vi "DisplayConsole_Main.vi"(8 "error in (no error)":errorcluster) -> (0 "error out":errorcluster)   [LabVIEW 2017]
doc: "This is Top Level VI for Display Console Module. You can communicate with this module using its API. Communication is made based on queue. This module has not User Interface so I chase State Machine architecture."
uses:
  General/Controls/#TD_General_CommunicationQueueStates_Enum.ctl
  Private controls/#TD_DisplayConsole_InnerData_Cluster.ctl
  Private controls/#TD_DisplayConsole_ModuleStates_Enum.ctl
  Private controls/#TD_DisplayConsole_ModuleData_Cluster.ctl
  General/Controls/#TD_General_FromWho_Enum.ctl
panel:
  out "CardRead":bool caption="Card Read"
  out "MessageScreen":string caption="Message Screen"
  out "CurrentTransaction":string caption="Current Transaction"
  # "[Covers: UI3]"
  # "[Covers: UI3A] \n[Covers: UI3B] \n[Covers: UI3C]"
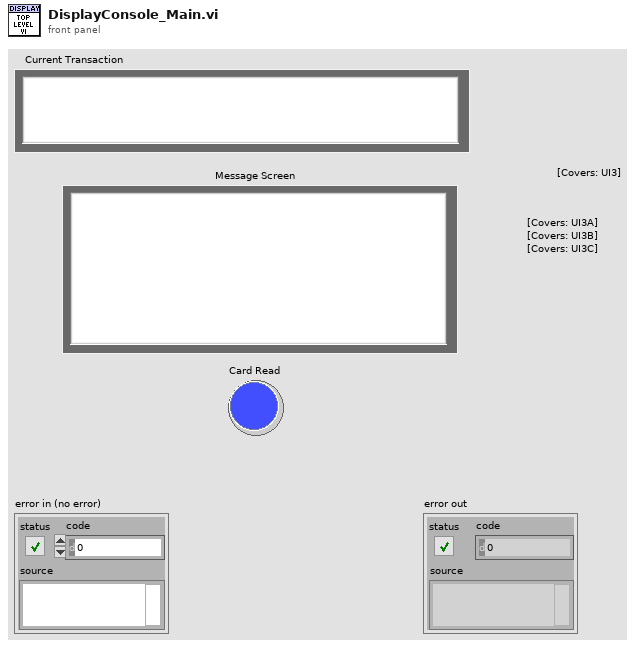
[diagram p1: front panel]
types:
  T1 = typedef "#TD_General_CommunicationQueueStates_Enum.ctl" = enum16{"ERROR_Default", "Obtain", "GetRef", "Enqueue", "EnqueueAtOpp", "GetStatus", "Release"}
  T2 = typedef "#TD_General_FromWho_Enum.ctl" = enum16{"ERROR_Default", "UserConsole", "DisplayConsole", "SensorInterface", "Controller", "Database", "Timing", "AdditionalModule", "ErrorHandling"}
  T3 = typedef "#TD_DisplayConsole_ModuleStates_Enum.ctl" = enum16{"ERROR_Default", "Init", "Close", "ErrorHandling", "UpdateCurrTrans", "UpdateMessage", "NewState", "UpdateCardRead"}
  T4 = typedef "#TD_DisplayConsole_ModuleData_Cluster.ctl" = cluster{"Action":T3, "Data":variant}
  T5 = typedef "#TD_General_IntermoduleData_Cluster.ctl" = cluster{"Sender":T2, "ModuleData":variant}
  T6 = typedef "#TD_DisplayConsole_InnerData_Cluster.ctl" = cluster{"Sth":bool, "CurrentTrans":string, "CardRead":bool, "Messages":string[], "NumericTestAK":dbl}
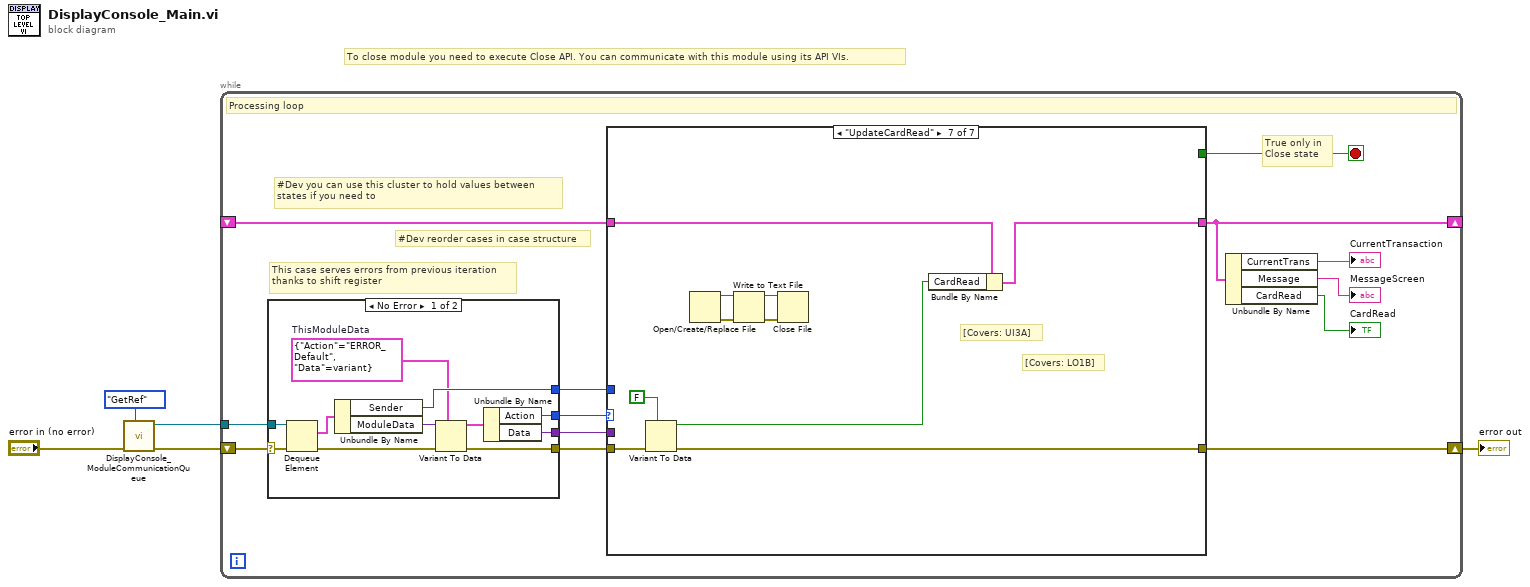
[diagram p0: block diagram]
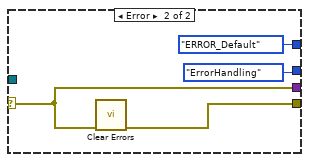
[diagram p2: hidden frame]
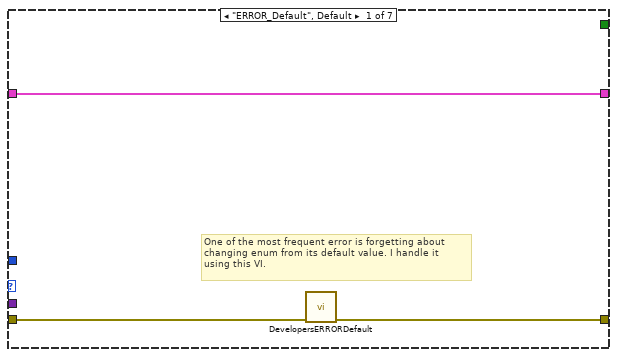
[diagram p3: hidden frame]
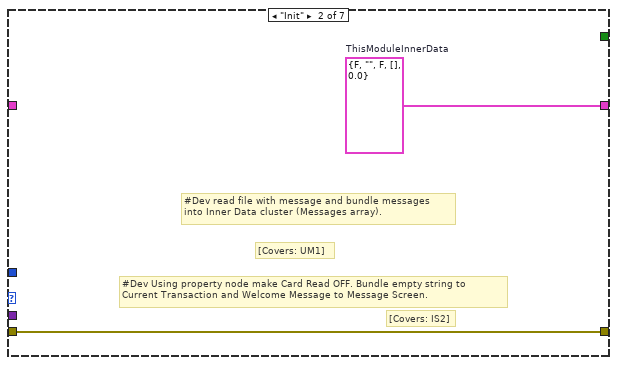
[diagram p4: hidden frame]
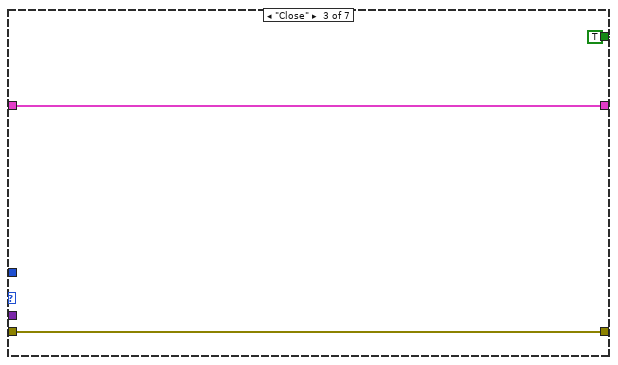
[diagram p5: hidden frame]
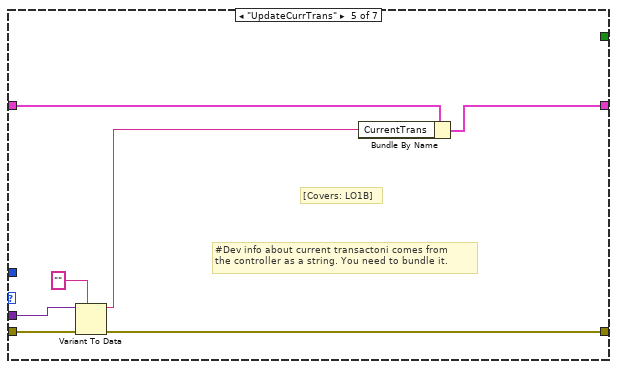
[diagram p7: hidden frame]
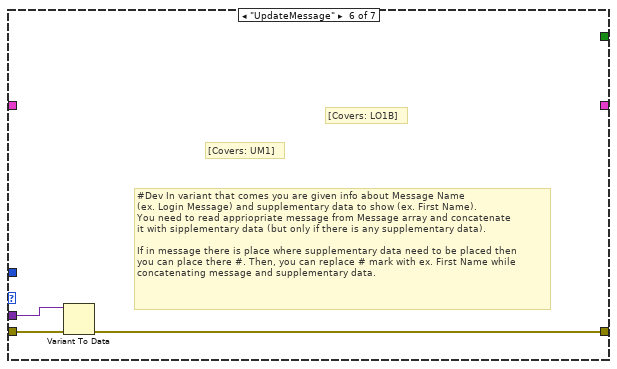
[diagram p8: hidden frame]
diagram:
  # "To close module you need to execute Close API. You can communicate with this module using its API VIs."
  n1 = call "DisplayConsole_ModuleCommunicationQueue.vi"("Action"=#TD_General_CommunicationQueueStates_Enum."GetRef", "error in (no error)"="error in (no error)") -> ("error out"=w2:errorcluster, "Ref out"=w3:refnum<queue>)  [unwired: 7 in, 1 out]
  n2 = while {
    tunnel: w3 -> [w17]
    shift-right: [w11] -> w1
    shift-left: w2 -> [w18]
    shift-right: [w9] -> _
    shift-left: _ -> [w16]
    stop <- w10 stop-if-true
    # "#Dev reorder cases in case structure"
    # "True only in \nClose state"
    # "#Dev you can use this cluster to hold values between \nstates if you need to"
    # "This case serves errors from previous iteration \nthanks to shift register"
    # "Processing loop"
    n3 = case shown="No Error" w18 {
      selector: w18 -> [w29 w33]
      tunnel: w17 -> [w28 _]
      tunnel: [w24 #TD_General_FromWho_Enum."ERROR_Default" ("Sender")] -> w15
      tunnel: [w21 #TD_DisplayConsole_ModuleStates_Enum."ErrorHandling" ("Action")] -> w14
      tunnel: [w20 w33] -> w13
      tunnel: [w19 w32] -> w12
      frame No Error {
        w23 = T4 {"Action"=enum."ERROR_Default", "Data"=variant}  # ThisModuleData
        n4 = Dequeue Element(queue=w28, error in (no error)=w29) -> (element=w27:T5, error out=w25:errorcluster)  [unwired: 1 in, 2 out]
        n5 = Unbundle By Name(w27) -> ("Sender"=w24:T2, "ModuleData"=w26:variant)
        n6 = Variant To Data(error in=w25, type=w23, Variant=w26) -> (data=w22:T4, error out=w19:errorcluster)
        n7 = Unbundle By Name(w22) -> ("Action"=w21:T3, "Data"=w20:variant)
      }
      frame Error {
        n8 = call <vilib>:"Clear Errors.vi"("error in (no error)"=w33) -> ("error out"=w32:errorcluster)  [unwired: 5 in, 1 out]
      }
    }
    n9 = case shown="\"UpdateCardRead\"" w14 {
      tunnel: [w36 w38 w40 w43 w47 _ w60] -> w9
      tunnel: w16 -> [w36 _ w40 w43 w48 _ w61]
      tunnel: w15 -> [_ _ _ _ _ _ _]
      tunnel: w13 -> [_ _ _ _ w49 w52 _]
      tunnel: w12 -> [w35 w37 w39 w42 w50 w53 w63]
      tunnel: [w34 w37 w39 w42 w45 w51 w58] -> w11
      tunnel: [_ _ TRUE _ _ _ _] -> w10
      frame "ERROR_Default", Default {
        # "One of the most frequent error is forgetting about \nchanging enum from its default value. I handle it \nusing this VI."
        n10 = call "DevelopersERRORDefault.vi"("error in (no error)"=w35) -> ("error out"=w34:errorcluster)  [unwired: 10 in]
      }
      frame "Init" {
        w38 = T6 {"Sth"=FALSE, "CurrentTrans"="", "CardRead"=FALSE, "Messages"=[], "NumericTestAK"=0.0}  # ThisModuleInnerData
        # "[Covers: IS2]"
        # "#Dev Using property node make Card Read OFF. Bundle empty string to \nCurrent Transaction and Welcome Message to Message Screen."
        # "[Covers: UM1]"
        # "#Dev read file with message and bundle messages \ninto Inner Data cluster (Messages array)."
      }
      frame "Close" {
      }
      frame "ErrorHandling" {
        # "#Dev take some actions to handle the error \nand inform central Error Handling Module \nabout this error using Error Handling Module \nAPI"
      }
      frame "UpdateCurrTrans" {
        # "[Covers: LO1B]"
        # "#Dev info about current transactoni comes from \nthe controller as a string. You need to bundle it."
        n11 = Variant To Data(error in=w50, type="", Variant=w49) -> (data=w44:string, error out=w45:errorcluster)
        n12 = Bundle By Name(cluster=w48, "CurrentTrans"=w44) -> (w47:T6)
      }
      frame "UpdateMessage" {
        # "[Covers: LO1B]"
        # "[Covers: UM1]"
        # "#Dev In variant that comes you are given info about Message Name \n(ex. Login Message) and supplementary data to show (ex. First Name). \nYou need to read appriopriate message from Message array and concatenate \nit with sipplementary data (but only if there is any supplementary data). \n\nIf in message there is place where supplementary data need to be placed then \nyou can place there #. Then, you can replace # mark with ex. First Name while \nconcatenating message and supplementary data."
        n13 = Variant To Data(error in=w53, Variant=w52) -> (error out=w51:errorcluster)  [unwired: 1 in, 1 out]
      }
      frame "UpdateCardRead" {
        # "[Covers: LO1B]"
        # "[Covers: UI3A]"
        n14 = Variant To Data(error in=w63, type=FALSE) -> (data=w59:bool, error out=w58:errorcluster)  [unwired: 1 in]
        n15 = Open/Create/Replace File() -> (refnum out=w56:refnum<file>, error out=w57:errorcluster)  [unwired: 6 in, 1 out]
        n16 = Write to Text File(file (use dialog)=w56, error in=w57) -> (refnum out=w54:refnum<file>, error out=w55:errorcluster)  [unwired: 2 in, 1 out]
        n17 = Close File(refnum=w54, error in=w55) -> ()  [unwired: 2 out]
        n18 = Bundle By Name(cluster=w61, "CardRead"=w59) -> (w60:T6)
      }
    }
    n19 = Unbundle By Name(w9) -> ("CurrentTrans"=→"CurrentTransaction":string, "Message"=→"MessageScreen":string, "CardRead"=→"CardRead":bool)
  }
  "error out" <- w1
